vi "Read Vpmt.vi"(8 "error in (no error)":errorcluster, 11 "Update PMT Gains MSG in":refnum<class "Update PMT Gains MSG.lvclass">) -> (0 "error out":errorcluster, 2 "Vpmt":dbl[](array[numeric]), 3 "Update PMT Gains MSG out":refnum<class "Update PMT Gains MSG.lvclass">)   [LabVIEW 2014, in "eCRDS Library.lvlib" / "Update PMT Gains MSG.lvclass"]
uses:
  Update PMT Gains MSG.lvclass
  Update PMT Gains MSG.lvclass/Update PMT Gains MSG.ctl
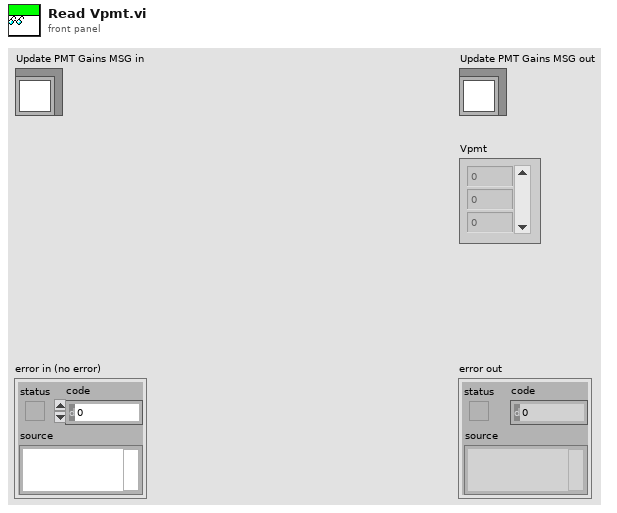
[diagram p1: front panel]
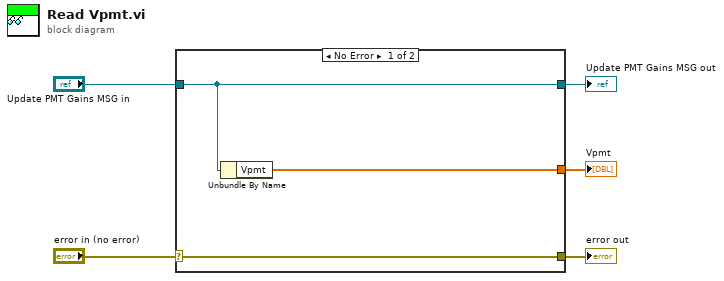
[diagram p0: block diagram]
diagram:
  n1 = case shown="No Error" "error in (no error)" {
    selector: "error in (no error)" -> [w8 w9]
    tunnel: [w8 w9] -> w4
    tunnel: [w7 w10] -> w2
    tunnel: "Update PMT Gains MSG in" -> [w7 w10]
    tunnel: [w6 _] -> w1
    frame No Error {
      n2 = Unbundle By Name(w7) -> ("Vpmt"=w6:dbl[])
    }
    frame Error {
    }
  }
  "error out" <- w4
  "Update PMT Gains MSG out" <- w2
  "Vpmt" <- w1
